vi "CameraControl_AsyncGrab.vi"() -> ()   [LabVIEW 2013]
uses:
  QImaging_Basic/Controls/Parameter.ctl
  Debug/QImaging.dll
panel:
  out "Camera Handle":u32
  in  "Abort Frame":bool
  out "sizeOfBuf":u32
  out "errcode":i32
  out "Queue frame err":i32
  out "pBuf address":u32
  out "pFrame address":u32
  out "Streaming error":i32
  out "streaming":bool
  in  "Streaming":bool
  in  "Grab Image":bool
  in  "Queue Frame":bool
  in  "Trig":bool
  out "Intensity Graph":u16[][](graph)
  out "CCD Height":u32=1 min=1 max=4 step=1
  out "CCD Width":u32=1 min=1 max=4 step=1
  in  "Binning":u32=1 min=1 max=4 step=1
  out "Open Cam Error":i32
  out "LibCam Error":u32
  out "LibOpen error":i32
  in  "Stop Camera":bool
  in  "Start Camera":bool
  in  "Exposure Time":u32=100
  out "ParamVal":u32[](array[numeric])
  out "Camera Id":u32
  out "error out":errorcluster
  in  "error in (no error)":errorcluster
  in  "Stop":bool
  # "Hardware"
  # "Freerun"
  # "Image Width"
  # "Image Height"
  # "Image Size"
  # "CCD Type"
  # "CCD Width"
  # "CCD Height"
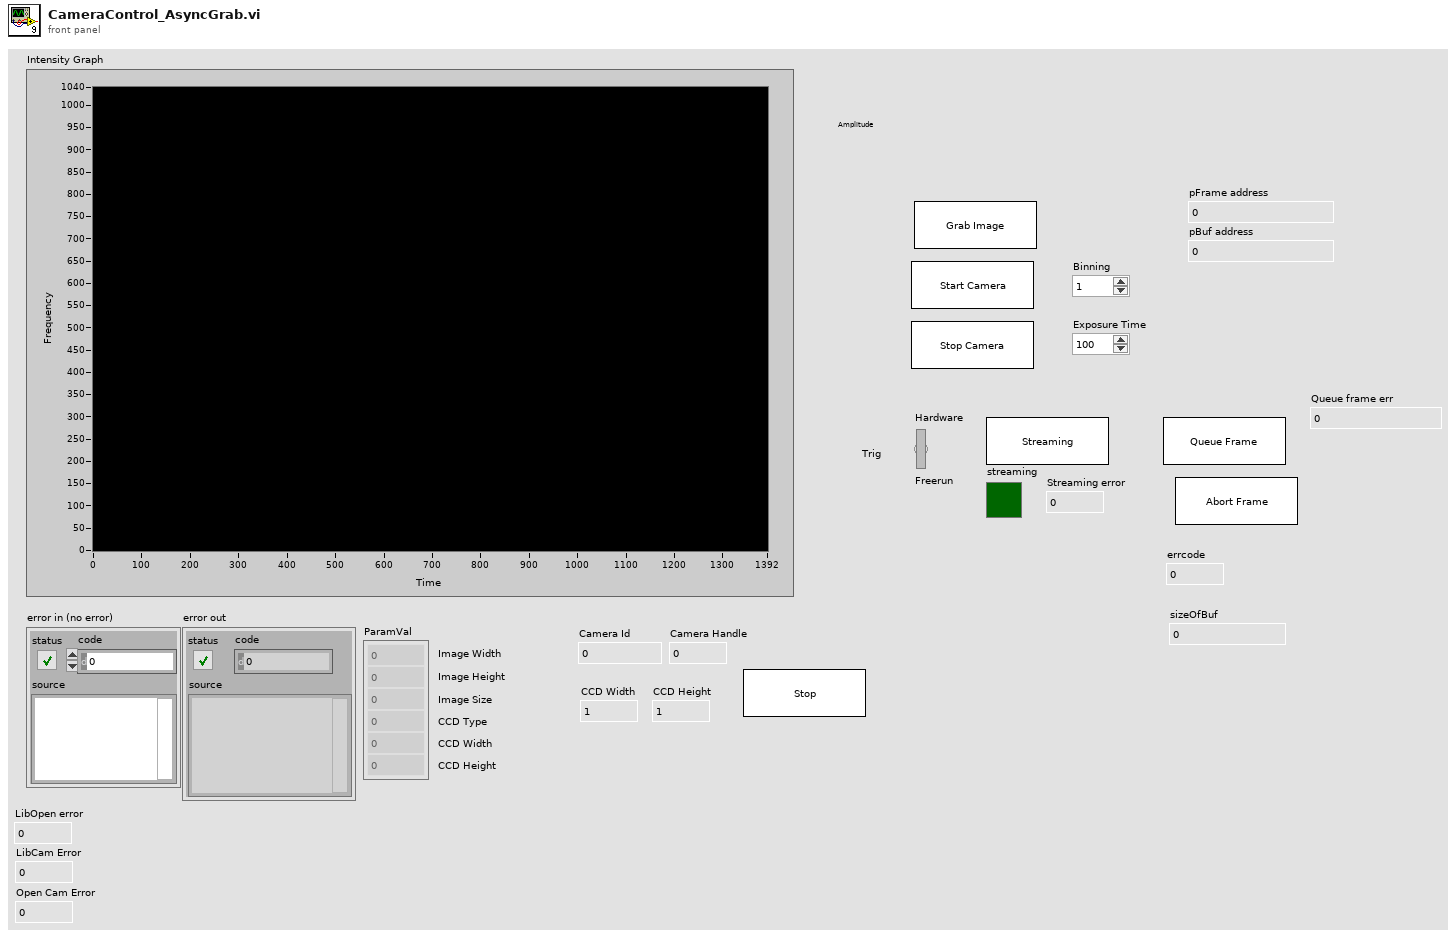
[diagram p1: front panel]
types:
  T1 = typedef "Parameter.ctl" = enum32{"Gain ", "Offset", "Exposure", "Binning", "HzBinning", "VtBinning", "Readout speed", "Trigger Type", "Color Wheel", "Cooler Active", "Exposure red", "Exposure blue", "Image format", "ROI X", "ROI Y", "ROI Width", "ROI Height"}
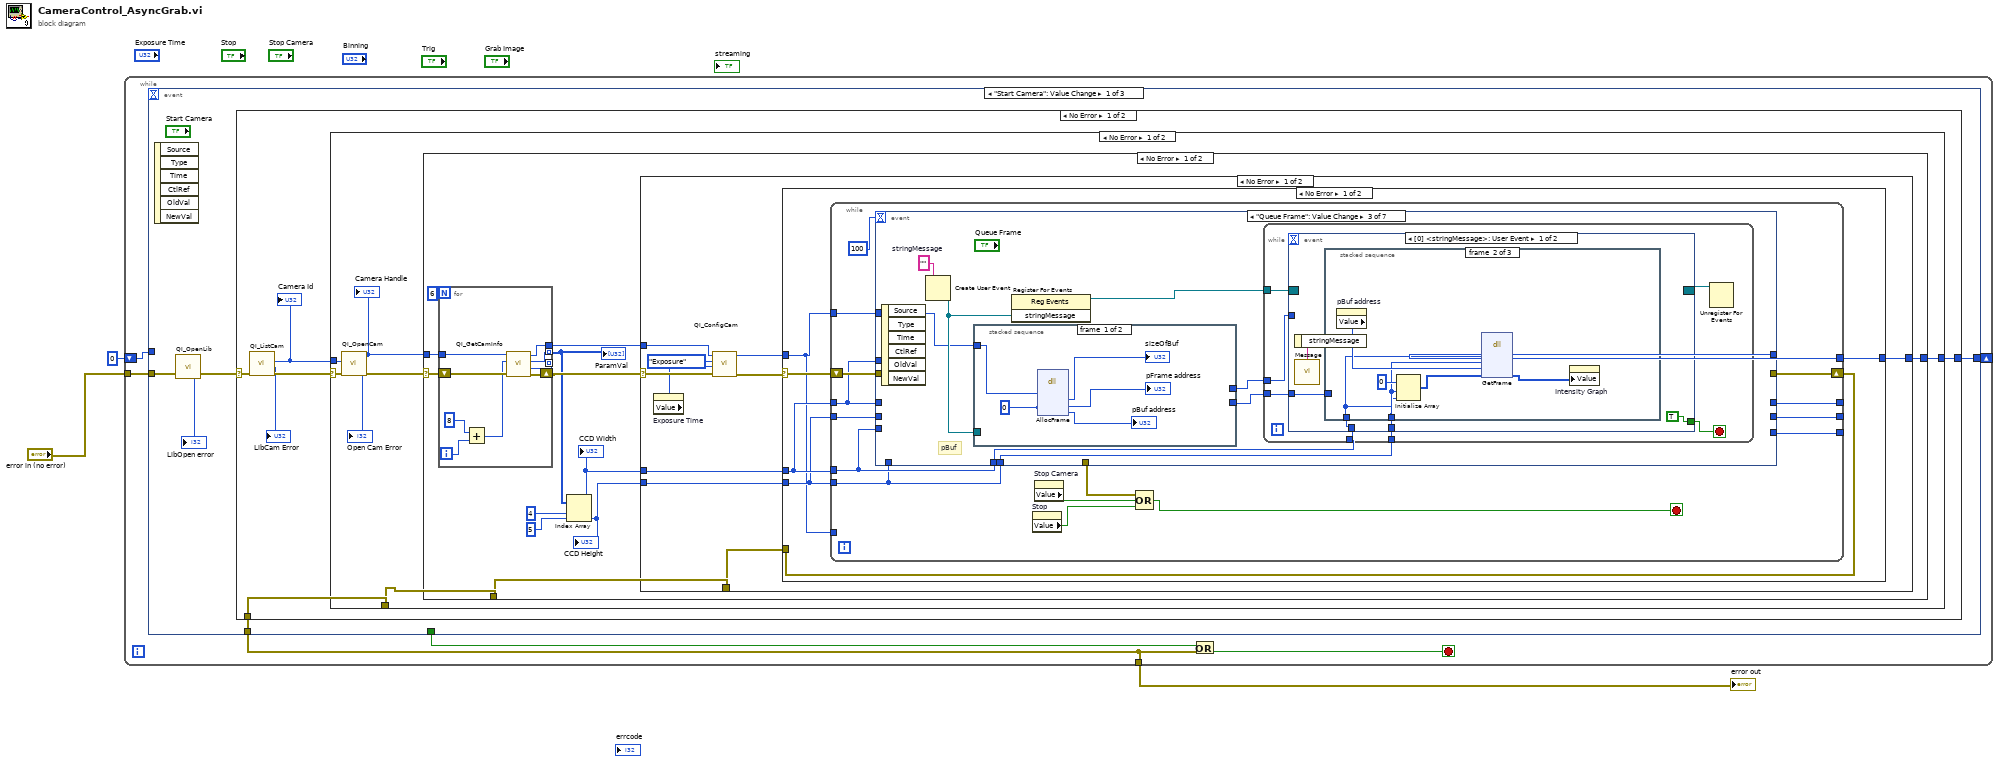
[diagram p0: block diagram]
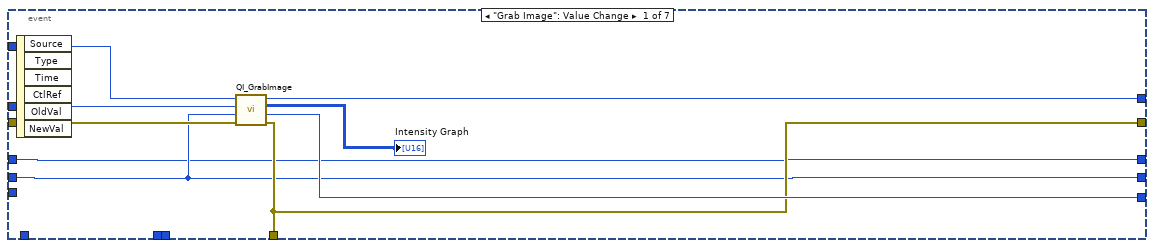
[diagram p2: hidden frame]
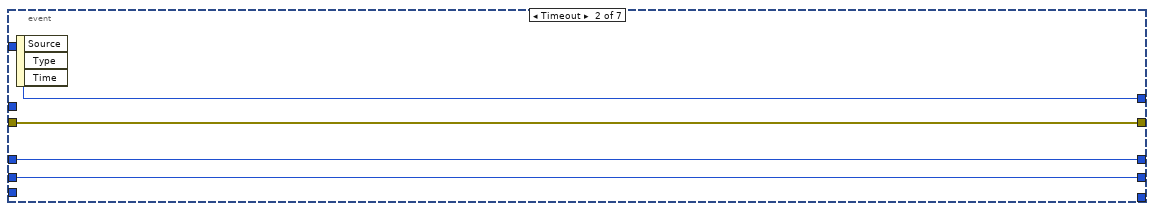
[diagram p3: hidden frame]
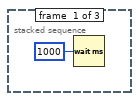
[diagram p4: hidden frame]
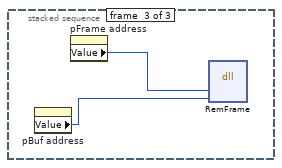
[diagram p5: hidden frame]
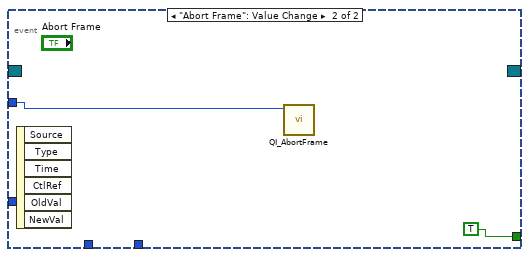
[diagram p6: hidden frame]
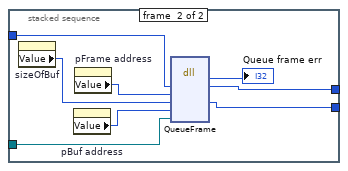
[diagram p7: hidden frame]
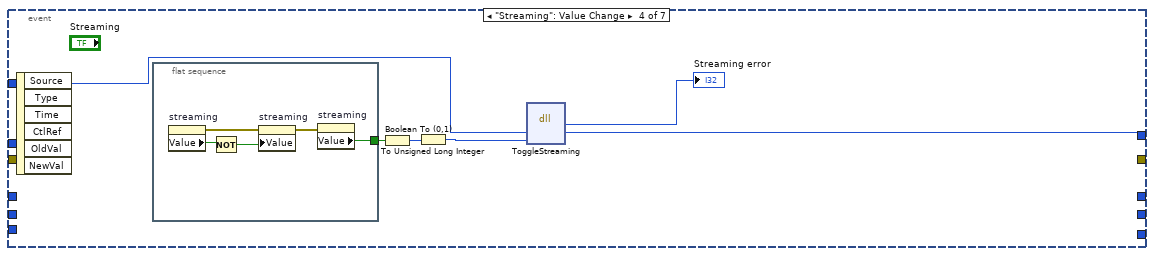
[diagram p8: hidden frame]
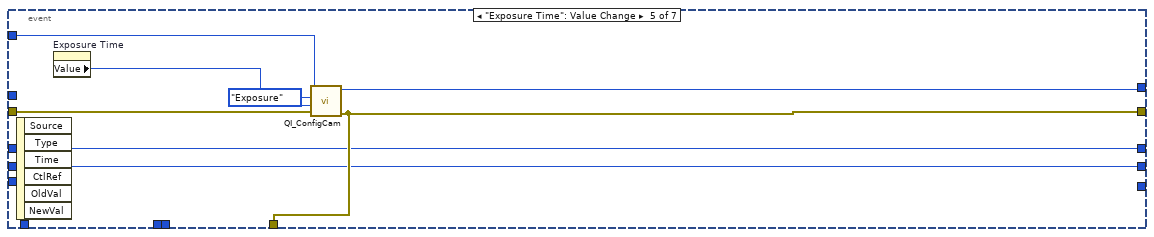
[diagram p9: hidden frame]
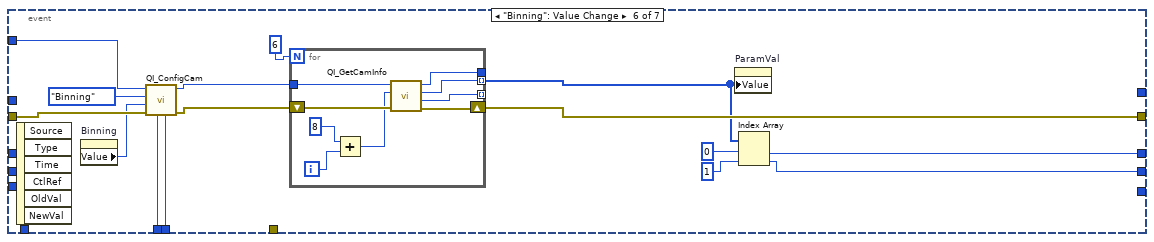
[diagram p10: hidden frame]
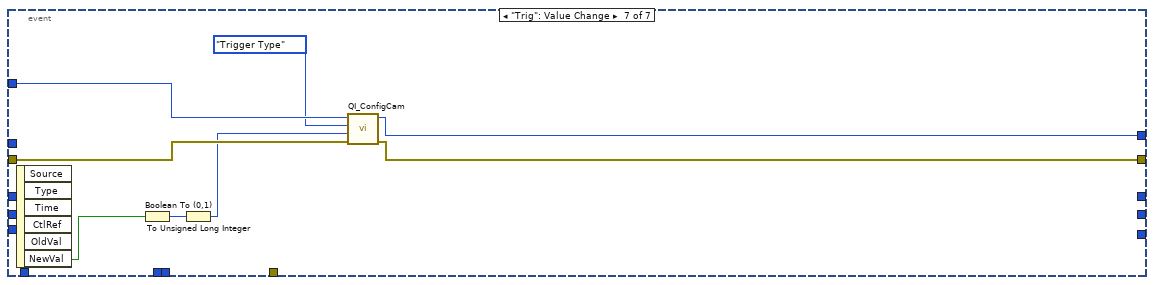
[diagram p11: hidden frame]
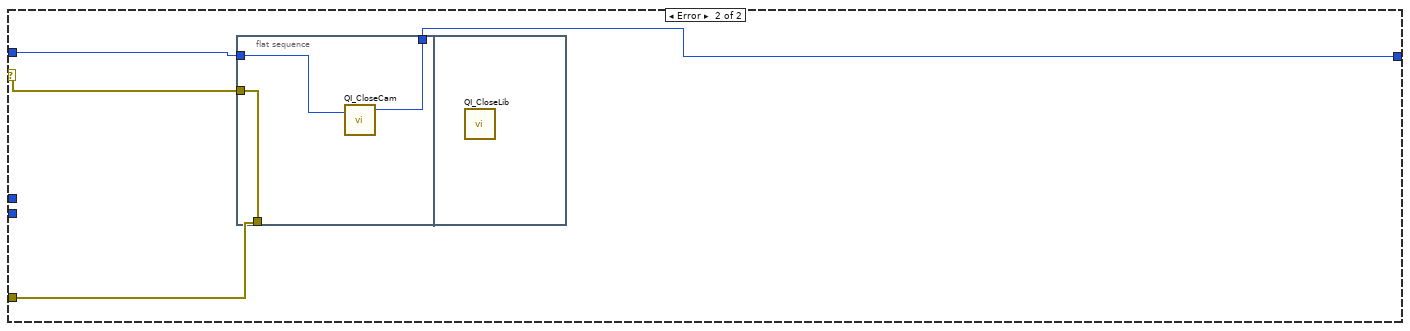
[diagram p12: hidden frame]
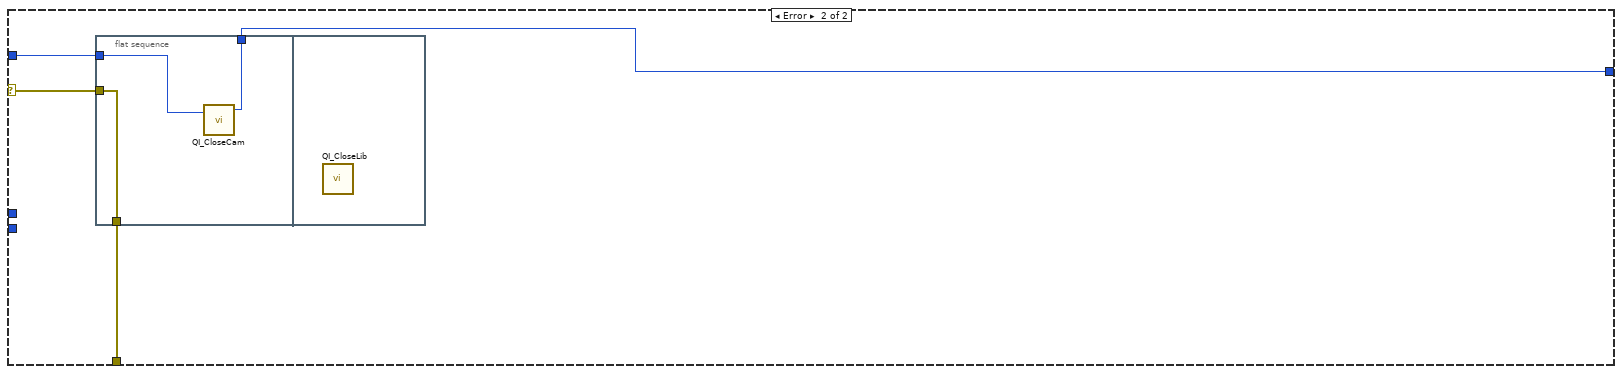
[diagram p13: hidden frame]
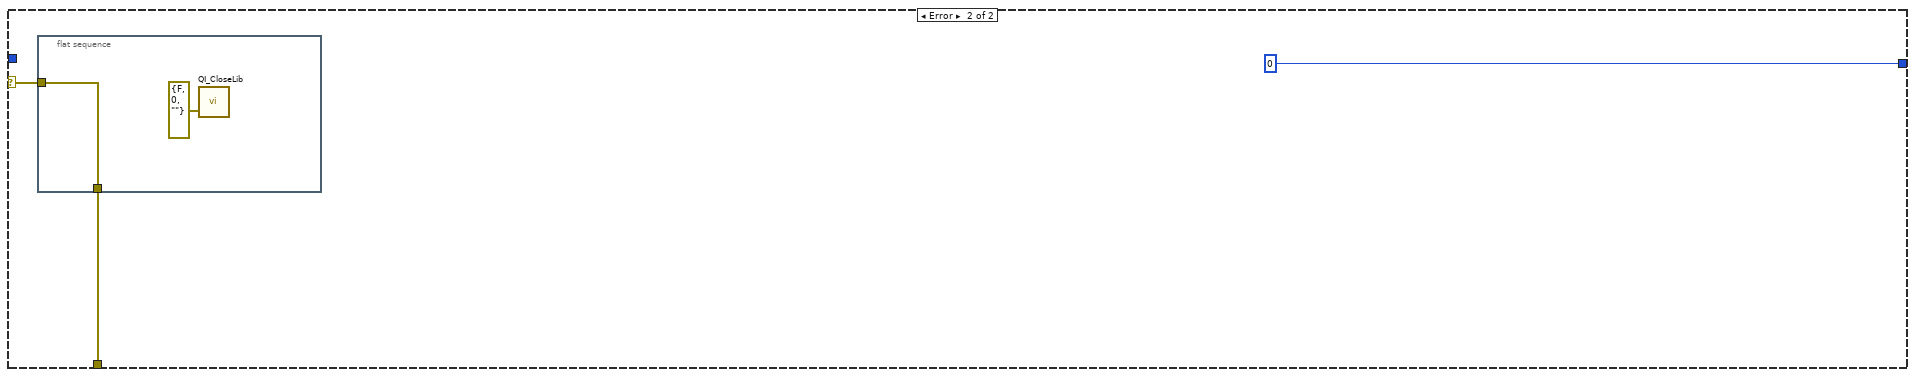
[diagram p14: hidden frame]
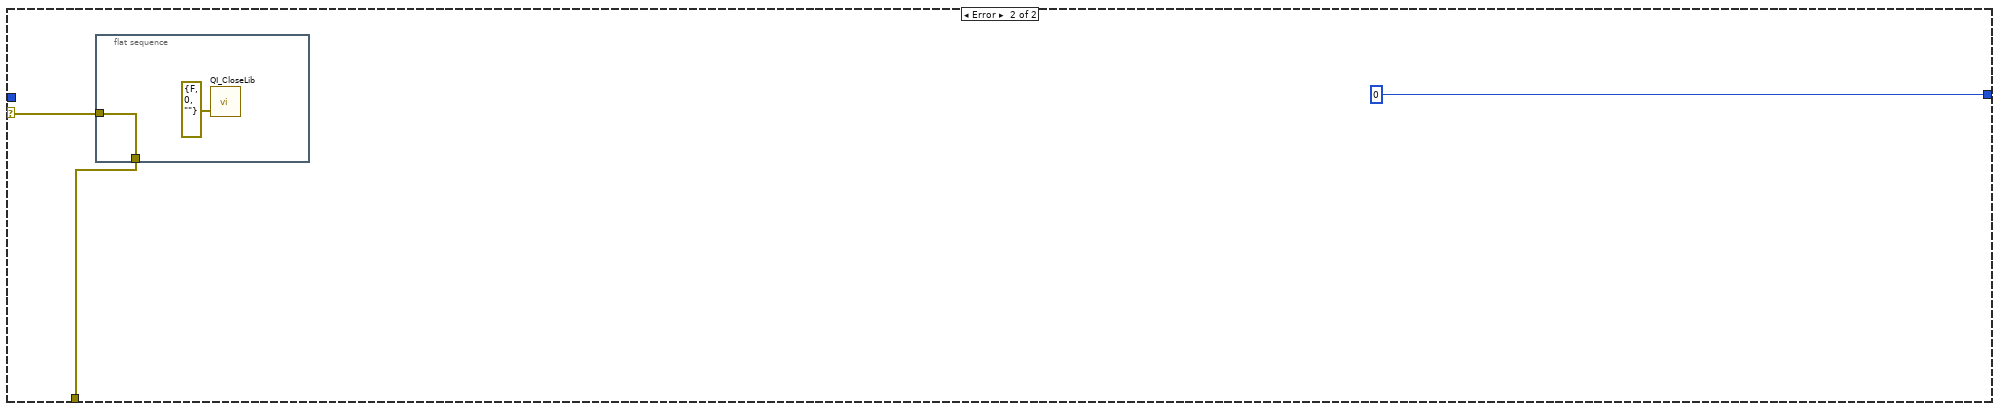
[diagram p15: hidden frame]
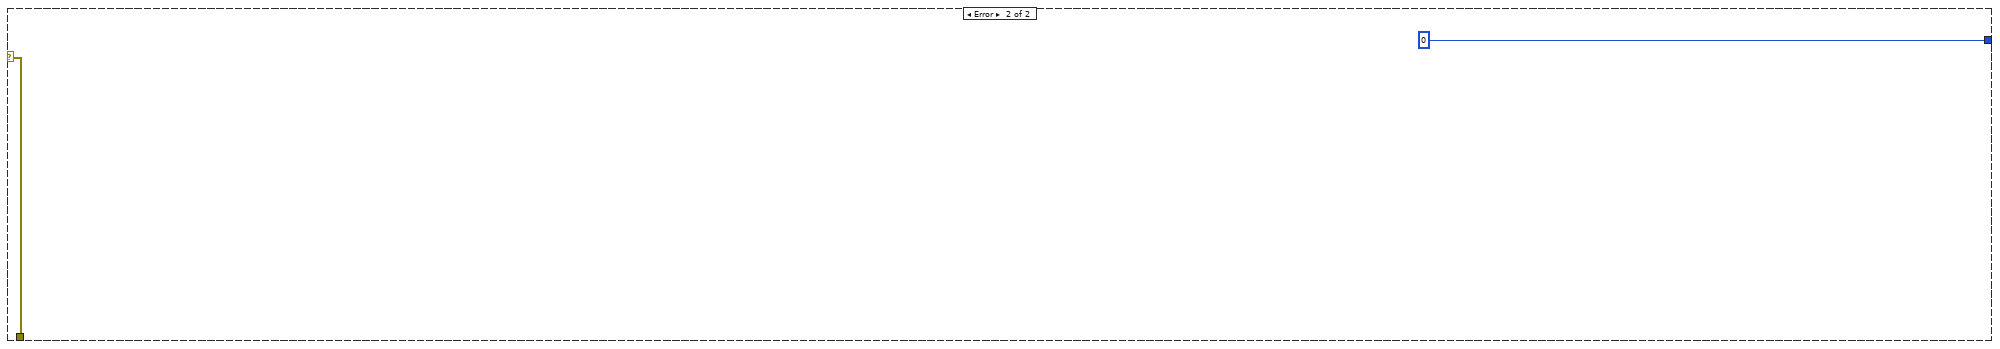
[diagram p16: hidden frame]
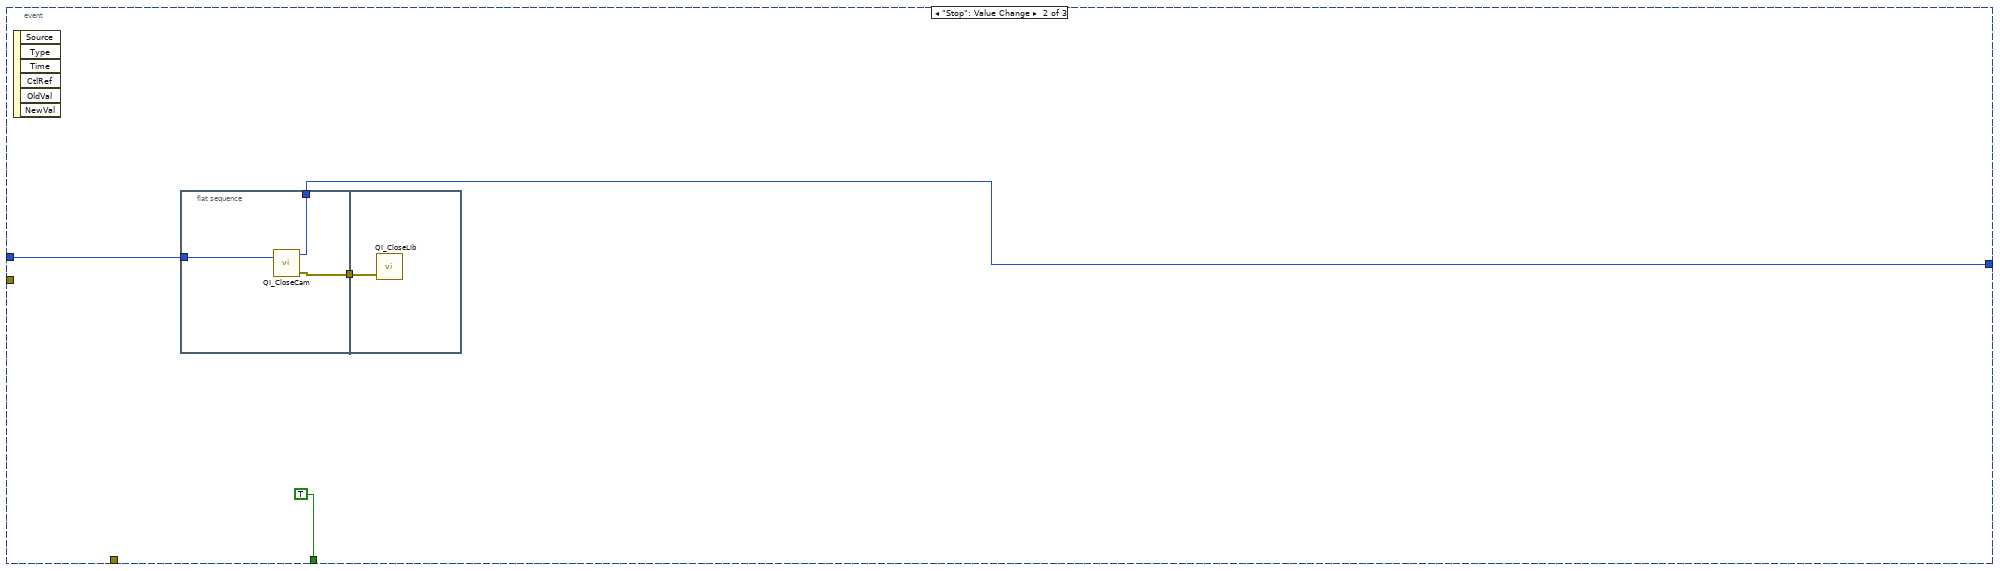
[diagram p17: hidden frame]
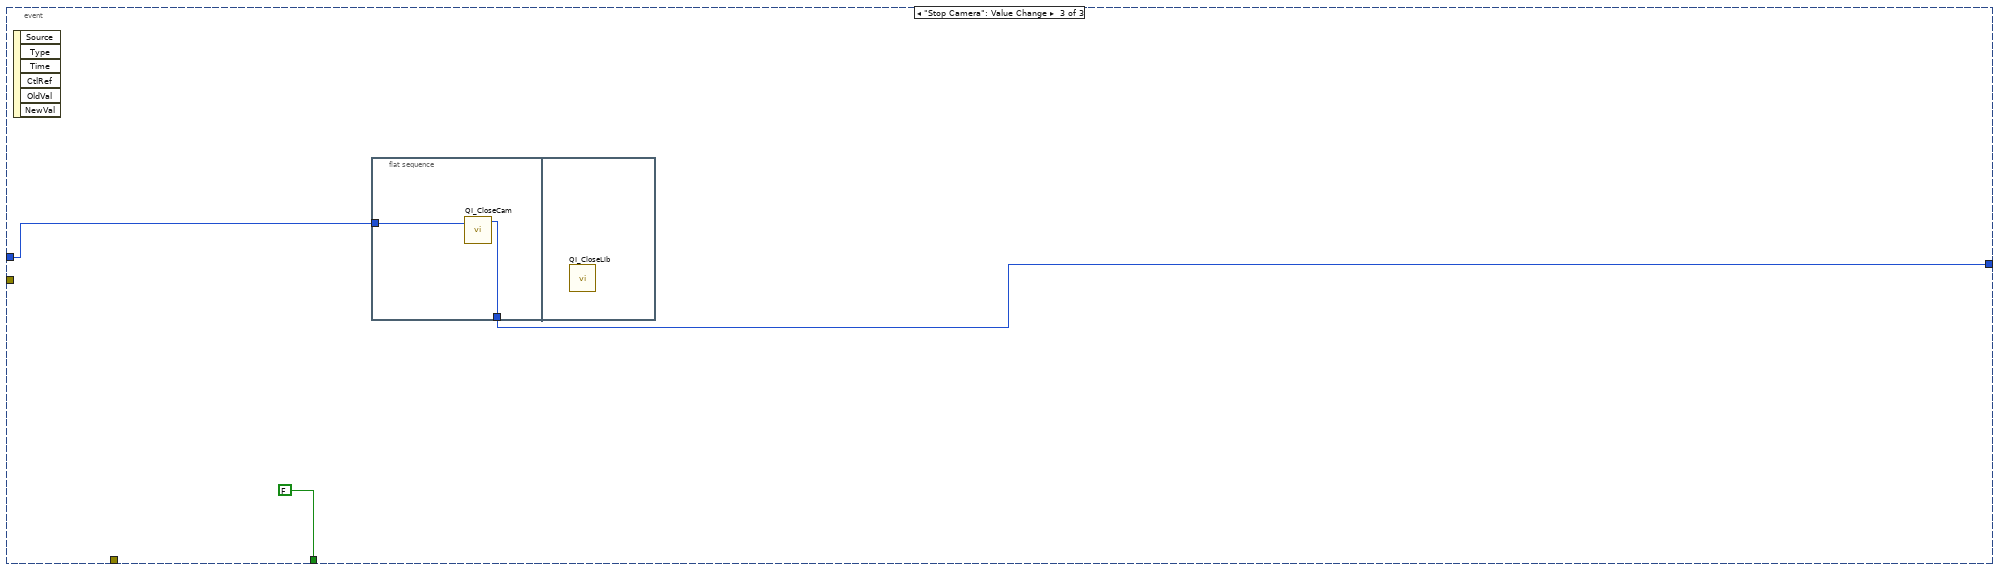
[diagram p18: hidden frame]
diagram:
  n1 = while {
    tunnel: "error in (no error)" -> [w9]
    shift-right: [w7] -> _
    shift-left: u32 0 ("Camera Handle") -> [w6]
    tunnel: [w5] -> w1
    stop <- w4 stop-if-true
    n2 = event shown="[0] \"Start Camera\": Value Change" {
      selector: _ -> [_ _ _]
      dyn-events: _ -> [_ _ _]
      timeout: _ -> [_ _ _]
      tunnel: w9 -> [w14 _ _]
      tunnel: [w12 _ _] -> w5
      tunnel: [_ TRUE FALSE] -> w8
      tunnel: [w11 w215 w223] -> w7
      tunnel: w6 -> [_ w217 w225]
      event "Start Camera": Value Change {
        n3 = event-data() -> ()  [unwired: 1 in, 6 out]
        n4 = call "QI_OpenLib.vi"("error in (no error)"=w14) -> ("error out"=w13:errorcluster, "LibOpen error"=→"LibOpen error":i32)  [unwired: 1 in]
        n5 = case shown="No Error" w13 {
          selector: w13 -> [w20 w214]
          tunnel: [w17 w214] -> w12
          tunnel: [w16 u32 0 ("Camera Handle")] -> w11
          frame No Error {
            n6 = call "QI_ListCam.vi"("error in (no error)"=w20) -> ("error out"=w19:errorcluster, "LibCam Error"=→"LibCam Error":u32, "cameraId"=w18:u32)  [unwired: 8 in]
            "Camera Id" <- w18
            n7 = case shown="No Error" w19 {
              selector: w19 -> [w27 w210]
              tunnel: w18 -> [w26 _]
              tunnel: [w24 w209] -> w17
              tunnel: [w23 u32 0 ("Camera Handle")] -> w16
              frame No Error {
                n8 = call "QI_OpenCam.vi"("error in (no error)"=w27, "Camera ID"=w26) -> ("error out"=w25:errorcluster, "Open Cam Error"=→"Open Cam Error":i32, "Camera Handle"=w21:u32)  [unwired: 7 in]
                "Camera Handle" <- w21
                n9 = case shown="No Error" w25 {
                  selector: w25 -> [w39 w205]
                  tunnel: w21 -> [w38 _]
                  tunnel: [w34 w204] -> w24
                  tunnel: [w33 u32 0 ("Camera Handle")] -> w23
                  frame No Error {
                    n10 = for {
                      N: 6 -> [_]
                      tunnel: w38 -> [w201]
                      shift-right: [w197] -> w36
                      shift-left: w39 -> [w202]
                      tunnel: [w196] -> w35
                      tunnel: [w195] -> w32 mode=indexing
                      tunnel: [w194] -> _ mode=indexing
                      i -> [w200]
                      n11 = Add(x=u32 8, y=w200) -> (x+y=w198:u32)
                      n12 = call "QI_GetCamInfo.vi"("error in (no error)"=w202, "paramKey"=w198, "Camera Handle"=w201) -> ("error out"=w197:errorcluster, "CamInfo err"=w194:i32, "paramVal"=w195:u32, "Camera Handle"=w196:u32)  [unwired: 5 in]
                    }
                    "ParamVal" <- w32
                    n13 = Index Array(array=w32, index #1=4 ("index"), index #2=5 ("index")) -> (element #1=w29:u32, element #2=w28:u32)
                    "CCD Width" <- w29
                    "CCD Height" <- w28
                    n14 = case shown="No Error" w36 {
                      selector: w36 -> [w49 w190]
                      tunnel: w35 -> [w48 w188]
                      tunnel: [w44 w189] -> w34
                      tunnel: [w43 w187] -> w33
                      tunnel: w29 -> [w41 _]
                      tunnel: w28 -> [w40 _]
                      frame No Error {
                        n15 = property on="Exposure Time" class="DigNum (strict)"() -> ("Value"=w47:u32)  [unwired: 2 in, 2 out]
                        n16 = call "QI_ConfigCam.vi"("error in (no error)"=w49, "paramVal"=w47, "Parameter"=Parameter."Exposure", "Camera Handle"=w48) -> ("error out"=w45:errorcluster, "Camera Handle"=w46:u32)  [unwired: 5 in, 1 out]
                        n17 = case shown="No Error" w45 {
                          selector: w45 -> [w55 w182]
                          tunnel: w46 -> [w50 w183]
                          tunnel: w41 -> [w52 _]
                          tunnel: w40 -> [w51 _]
                          tunnel: [w53 w181] -> w44
                          tunnel: [w54 w180] -> w43
                          frame No Error {
                            n18 = while {
                              tunnel: w50 -> [w71]
                              tunnel: [w67] -> _
                              tunnel: [w65] -> w54
                              shift-right: [w64] -> w53
                              shift-left: w55 -> [w70]
                              tunnel: w52 -> [w58]
                              tunnel: w51 -> [w57]
                              tunnel: w52 -> [w60]
                              tunnel: [w63] -> _
                              tunnel: w51 -> [w61]
                              tunnel: [w62] -> _
                              tunnel: w50 -> [_]
                              stop <- w56 stop-if-true
                              n19 = event shown="[2] \"Queue Frame\": Value Change" {
                                selector: _ -> [_ _ _ _ _ _ _]
                                dyn-events: _ -> [_ _ _ _ _ _ _]
                                timeout: 100 -> [_ _ _ _ _ _ _]
                                tunnel: w71 -> [w80 w84 w86 w131 w147 w162 w179]
                                tunnel: w70 -> [w79 w83 _ _ w144 w160 w176]
                                tunnel: w60 -> [w78 _ _ _ _ _ _]
                                tunnel: [w75 _ _ _ w143 _ _] -> w69
                                tunnel: [w77 w84 _ w130 w146 _ w178] -> w65
                                tunnel: [w76 _ _ _ _ _ _] -> w67
                                tunnel: [w75 w83 _ _ w143 w159 w177] -> w64
                                tunnel: [w73 w82 _ _ w142 w155 _] -> w63
                                tunnel: [w74 w81 _ _ w141 w154 _] -> w62
                                tunnel: w61 -> [w74 w81 _ _ w141 _ _]
                                tunnel: w60 -> [w73 w82 _ _ w142 _ _]
                                tunnel: w58 -> [_ _ w88 _ _ w149 _]
                                tunnel: w57 -> [_ _ w87 _ _ w148 _]
                                tunnel: w58 -> [_ _ _ _ _ _ _]
                                tunnel: w57 -> [_ _ _ _ _ _ _]
                                event "Grab Image": Value Change {
                                n20 = event-data() -> ()  [unwired: 1 in, 6 out]
                                n21 = call "QI_GrabImage.vi"("error in (no error)"=w79, "Image Width"=w74, "Image Height"=w78, "Camera Handle"=w80) -> ("error out"=w75:errorcluster, "GrabImage err"=w76:u32, "data"=→"Intensity Graph":u16[][], "Camera Handle"=w77:u32)  [unwired: 4 in]
                                }
                                event Timeout {
                                n22 = event-data() -> ()  [unwired: 1 in, 3 out]
                                }
                                event "Queue Frame": Value Change {
                                w92 = ""  # stringMessage
                                # "pBuf"
                                n23 = event-data() -> ()  [unwired: 1 in, 6 out]
                                n24 = Create User Event(user event datatype=w92) -> (user event=w91:refnum<user-event>)  [unwired: 1 in, 1 out]
                                n25 = stacked-sequence {
                                tunnel: w91 -> [_ w128]
                                tunnel: w86 -> [w119 w125]
                                tunnel: [_ w123] -> w89
                                tunnel: [_ w121] -> w85
                                frame #0 {
                                w120 = u32 0 ("pBuf")
                                n26 = dll-call lib="C:/Users/vernier/Documents/Visual Studio 2012/Projects/QImaging/Debug/QImaging.dll" fn="AllocFrame"("handle"=w119, "sizeOfBuf"=w120, "pFrame"=w120, "pBuf"=w120) -> ("sizeOfBuf"=→"sizeOfBuf":u32, "pFrame"=→"pFrame address":u32, "pBuf"=→"pBuf address":u32)  [unwired: 5 in, 2 out]
                                }
                                frame #1 {
                                n27 = property on="sizeOfBuf" class="DigNum (strict)"() -> ("Value"=w124:u32)  [unwired: 2 in, 2 out]
                                n28 = property on="pBuf address" class="DigNum (strict)"() -> ("Value"=w126:u32)  [unwired: 2 in, 2 out]
                                n29 = property on="pFrame address" class="DigNum (strict)"() -> ("Value"=w127:u32)  [unwired: 2 in, 2 out]
                                n30 = dll-call lib="C:/Users/vernier/Documents/Visual Studio 2012/Projects/QImaging/Debug/QImaging.dll" fn="QueueFrame"("handle"=w125, "pFrame"=w127, "bufferSize"=w124, "pBuf"=w126, "UserEventRef"=w128) -> ("return type"=→"Queue frame err":i32, "handle"=w121:u32, "bufferSize"=w123:u32)  [unwired: 6 in, 2 out]
                                }
                                }
                                n31 = register-events(w91) -> (reference out=w90:refnum<event-registration>)  [unwired: 2 in, 1 out]
                                n32 = while {
                                tunnel: w90 -> [w99]
                                tunnel: w89 -> [w98]
                                tunnel: w88 -> [w97]
                                tunnel: w87 -> [w96]
                                tunnel: w85 -> [w94]
                                stop <- w93 stop-if-true
                                n33 = event shown="[0] <stringMessage>: User Event" {
                                selector: w99 -> [_ _]
                                dyn-events: [_ _] -> w95
                                timeout: _ -> [_ _]
                                tunnel: w98 -> [w103 _]
                                tunnel: w97 -> [w102 _]
                                tunnel: w96 -> [w101 _]
                                tunnel: [TRUE TRUE] -> w93
                                tunnel: w94 -> [_ w114]
                                event User Event {
                                n34 = event-data() -> ("stringMessage"=w104:string)  [unwired: 1 in]
                                n35 = call "Message.vi"("String"=w104) -> ()
                                n36 = stacked-sequence {
                                tunnel: w103 -> [_ _ _]
                                tunnel: w102 -> [_ w106 _]
                                tunnel: w101 -> [_ w107 _]
                                frame #0 {
                                n37 = Wait (ms)(milliseconds to wait=u32 1000) -> ()  [unwired: 1 out]
                                }
                                frame #1 {
                                n38 = property on="pBuf address" class="DigNum (strict)"() -> ("Value"=w111:u32)  [unwired: 2 in, 2 out]
                                n39 = Initialize Array(u16 0 ("element"), w107, w106) -> (w109:u16[][])
                                n40 = dll-call lib="C:/Users/vernier/Documents/Visual Studio 2012/Projects/QImaging/Debug/QImaging.dll" fn="GetFrame"("width"=w106, "height"=w107, "pBuf"=w111, "data"=w109) -> ("data"=w108:u16[][])  [unwired: 7 in, 2 out]
                                n41 = property on="Intensity Graph" class="IntGraph (strict)"("Value"=w108) -> ()  [unwired: 2 in, 2 out]
                                }
                                frame #2 {
                                n42 = property on="pBuf address" class="DigNum (strict)"() -> ("Value"=w112:u32)  [unwired: 2 in, 2 out]
                                n43 = property on="pFrame address" class="DigNum (strict)"() -> ("Value"=w113:u32)  [unwired: 2 in, 2 out]
                                n44 = dll-call lib="C:/Users/vernier/Documents/Visual Studio 2012/Projects/QImaging/Debug/QImaging.dll" fn="RemFrame"("pFrame"=w113, "pBuf"=w112) -> ()  [unwired: 6 in, 2 out]
                                }
                                }
                                }
                                event "Abort Frame": Value Change {
                                n45 = event-data() -> ()  [unwired: 1 in, 6 out]
                                n46 = call "QI_AbortFrame.vi"("Camera Handle"=w114) -> ()  [unwired: 9 in, 2 out]
                                }
                                }
                                n47 = Unregister For Events(event registration refnum=w95) -> ()  [unwired: 1 in, 1 out]
                                }
                                }
                                event "Streaming": Value Change {
                                n48 = event-data() -> ()  [unwired: 1 in, 6 out]
                                n49 = flat-sequence {
                                tunnel: [w135] -> w132
                                frame #0 {
                                n50 = property on="streaming" class="Bool (strict)"() -> (error out=w139:errorcluster, "Value"=w138:bool)  [unwired: 2 in, 1 out]
                                n51 = Not(x=w138) -> (.not. x?=w137:bool)
                                n52 = property on="streaming" class="Bool (strict)"(error in=w139, "Value"=w137) -> (error out=w136:errorcluster)  [unwired: 1 in, 1 out]
                                n53 = property on="streaming" class="Bool (strict)"(error in=w136) -> ("Value"=w135:bool)  [unwired: 1 in, 2 out]
                                }
                                }
                                n54 = Boolean To (0,1)(Boolean=w132) -> (0, 1=w134:i16)
                                n55 = To Unsigned Long Integer(number=w134) -> (unsigned 32bit integer=w133:u32)
                                n56 = dll-call lib="C:/Users/vernier/Documents/Visual Studio 2012/Projects/QImaging/Debug/QImaging.dll" fn="ToggleStreaming"("handle"=w131, "enable"=w133) -> ("return type"=→"Streaming error":i32, "handle"=w130:u32)  [unwired: 4 in, 2 out]
                                }
                                event "Exposure Time": Value Change {
                                n57 = event-data() -> ()  [unwired: 1 in, 6 out]
                                n58 = property on="Exposure Time" class="DigNum (strict)"() -> ("Value"=w145:u32)  [unwired: 2 in, 2 out]
                                n59 = call "QI_ConfigCam.vi"("error in (no error)"=w144, "paramVal"=w145, "Parameter"=Parameter."Exposure", "Camera Handle"=w147) -> ("error out"=w143:errorcluster, "Camera Handle"=w146:u32)  [unwired: 5 in, 1 out]
                                }
                                event "Binning": Value Change {
                                n60 = event-data() -> ()  [unwired: 1 in, 6 out]
                                n61 = property on="Binning" class="DigNum (strict)"() -> ("Value"=w152:u32)  [unwired: 2 in, 2 out]
                                n62 = call "QI_ConfigCam.vi"("CCD Height"=w148, "CCD Width"=w149, "error in (no error)"=w160, "paramVal"=w152, "Parameter"=Parameter."Binning", "Camera Handle"=w162) -> ("error out"=w151:errorcluster, "Camera Handle"=w153:u32)  [unwired: 3 in, 1 out]
                                n63 = for {
                                N: 6 -> [_]
                                shift-right: [w167] -> w159
                                shift-left: w151 -> [w171]
                                tunnel: [w166] -> _
                                tunnel: [w165] -> w158 mode=indexing
                                tunnel: [w164] -> _ mode=indexing
                                tunnel: w153 -> [w163]
                                i -> [w170]
                                n64 = Add(x=u32 8, y=w170) -> (x+y=w168:u32)
                                n65 = call "QI_GetCamInfo.vi"("error in (no error)"=w171, "paramKey"=w168, "Camera Handle"=w163) -> ("error out"=w167:errorcluster, "CamInfo err"=w164:i32, "paramVal"=w165:u32, "Camera Handle"=w166:u32)  [unwired: 5 in]
                                }
                                n66 = property on="ParamVal" class="Arr (strict)"("Value"=w158) -> ()  [unwired: 2 in, 2 out]
                                n67 = Index Array(array=w158, index #1=0 ("index"), index #2=1 ("index")) -> (element #1=w155:u32, element #2=w154:u32)
                                }
                                event "Trig": Value Change {
                                n68 = event-data() -> ("NewVal"=w174:bool)  [unwired: 1 in, 5 out]
                                n69 = Boolean To (0,1)(Boolean=w174) -> (0, 1=w173:i16)
                                n70 = To Unsigned Long Integer(number=w173) -> (unsigned 32bit integer=w172:u32)
                                n71 = call "QI_ConfigCam.vi"("error in (no error)"=w176, "paramVal"=w172, "Parameter"=Parameter."Trigger Type", "Camera Handle"=w179) -> ("error out"=w177:errorcluster, "Camera Handle"=w178:u32)  [unwired: 5 in, 1 out]
                                }
                              }
                              n72 = property on="Stop" class="Bool (strict)"() -> ("Value"=w66:bool)  [unwired: 2 in, 2 out]
                              n73 = property on="Stop Camera" class="Bool (strict)"() -> ("Value"=w68:bool)  [unwired: 2 in, 2 out]
                              n74 = Compound Arithmetic op=OR(w69, w68, w66) -> (w56:bool)
                            }
                          }
                          frame Error {
                            n75 = flat-sequence {
                              tunnel: w182 -> [w185]
                              tunnel: [w185] -> w181
                              tunnel: w183 -> [w186]
                              tunnel: [w184] -> w180
                              frame #0 {
                                n76 = call "QI_CloseCam.vi"("Camera Handle"=w186) -> ("Camera Handle"=w184:u32)  [unwired: 1 in, 2 out]
                              }
                              frame #1 {
                                n77 = call "QI_CloseLib.vi"() -> ()  [unwired: 2 in, 2 out]
                              }
                            }
                          }
                        }
                      }
                      frame Error {
                        n78 = flat-sequence {
                          tunnel: w190 -> [w192]
                          tunnel: [w192] -> w189
                          tunnel: w188 -> [w193]
                          tunnel: [w191] -> w187
                          frame #0 {
                            n79 = call "QI_CloseCam.vi"("Camera Handle"=w193) -> ("Camera Handle"=w191:u32)  [unwired: 1 in, 2 out]
                          }
                          frame #1 {
                            n80 = call "QI_CloseLib.vi"() -> ()  [unwired: 2 in, 2 out]
                          }
                        }
                      }
                    }
                  }
                  frame Error {
                    n81 = flat-sequence {
                      tunnel: w205 -> [w207]
                      tunnel: [w207] -> w204
                      frame #0 {
                        n82 = call "QI_CloseLib.vi"("error in (no error)"=errorcluster {"status"=FALSE, "code"=0, "source"=""}) -> ()  [unwired: 1 in, 2 out]
                      }
                    }
                  }
                }
              }
              frame Error {
                n83 = flat-sequence {
                  tunnel: w210 -> [w212]
                  tunnel: [w212] -> w209
                  frame #0 {
                    n84 = call "QI_CloseLib.vi"("error in (no error)"=errorcluster {"status"=FALSE, "code"=0, "source"=""}) -> ()  [unwired: 1 in, 2 out]
                  }
                }
              }
            }
          }
          frame Error {
          }
        }
      }
      event "Stop": Value Change {
        n85 = event-data() -> ()  [unwired: 1 in, 6 out]
        n86 = flat-sequence {
          tunnel: w217 -> [w221]
          tunnel: [w220] -> w216
          tunnel: [w219] -> w215
          tunnel: w216 -> [w222]
          frame #0 {
            n87 = call "QI_CloseCam.vi"("Camera Handle"=w221) -> ("Camera Handle"=w219:u32, "error out"=w220:errorcluster)  [unwired: 1 in, 1 out]
          }
          frame #1 {
            n88 = call "QI_CloseLib.vi"("error in (no error)"=w222) -> ()  [unwired: 1 in, 2 out]
          }
        }
      }
      event "Stop Camera": Value Change {
        n89 = event-data() -> ()  [unwired: 1 in, 6 out]
        n90 = flat-sequence {
          tunnel: w225 -> [w227]
          tunnel: [w226] -> w223
          frame #0 {
            n91 = call "QI_CloseCam.vi"("Camera Handle"=w227) -> ("Camera Handle"=w226:u32)  [unwired: 1 in, 2 out]
          }
          frame #1 {
            n92 = call "QI_CloseLib.vi"() -> ()  [unwired: 2 in, 2 out]
          }
        }
      }
    }
    n93 = Or(x=w8, y=w5) -> (x .or. y?=w4:bool)
  }
  "error out" <- w1
